vi "Msg Q Alias.vi"(11 "Msg Q in":refnum<class "Msg Q.lvclass">) -> (0 "error out":errorcluster, 2 "Msg Q Alias":string)   [LabVIEW 2021, in "AAM.lvlib" / "Msg Q.lvclass"]
uses:
  Msg Q.lvclass
  Msg Q.lvclass/Msg Q.ctl
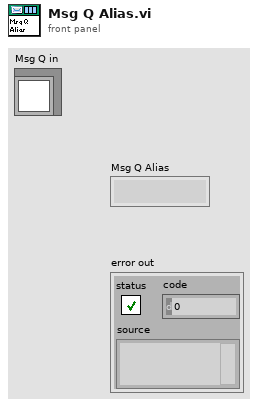
[diagram p1: front panel]
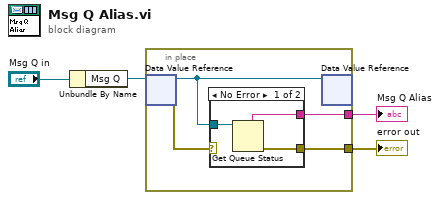
[diagram p0: block diagram]
diagram:
  n1 = Unbundle By Name("Msg Q in") -> ("Msg Q"=w4:refnum<data-value>)
  n2 = in-place {
    in-place-border: [w7] -> w3
    in-place-border: [w5] -> w1
    n3 = in-place-dvr #1(w4) -> (w6:refnum<queue>, w8:errorcluster)
    n4 = case shown="No Error" w8 {
      selector: w8 -> [_ w12]
      tunnel: w6 -> [w11 _]
      tunnel: [w10 w12] -> w7
      tunnel: [w9 _] -> w5
      frame No Error {
        n5 = Get Queue Status(queue=w11) -> (queue name=w9:string, error out=w10:errorcluster)  [unwired: 2 in, 6 out]
      }
      frame Error {
      }
    }
    n6 = in-place-dvr #1(w6) -> ()  [unwired: 2 out]
  }
  "error out" <- w3
  "Msg Q Alias" <- w1
